vi "DSF.Shared.Configuration.Transfer.Set Channel Configurations.vi"(10 "Channel Configurations":refnum<class "DSF.Shared.Configuration.Channel.lvclass">[](array[class]), 11 "Transfer Configuration in":refnum<class "DSF.Shared.Configuration.Transfer.lvclass">) -> (3 "Transfer Configuration out":refnum<class "DSF.Shared.Configuration.Transfer.lvclass">)   [LabVIEW 2016, in "DSF.Shared.lvlib" / "DSF.Shared.Configuration.Transfer.lvclass"]
uses:
  DSF.Shared.Configuration.Transfer.lvclass
  Channel/DSF.Shared.Configuration.Channel.lvclass
  DSF.Shared.Configuration.Transfer.lvclass/DSF.Shared.Configuration.Transfer.ctl
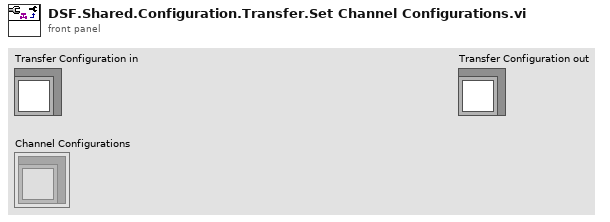
[diagram p1: front panel]
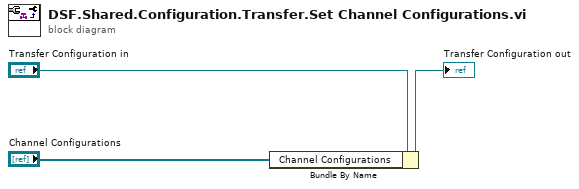
[diagram p0: block diagram]
diagram:
  n1 = Bundle By Name(cluster="Transfer Configuration in", "Channel Configurations"="Channel Configurations") -> (→"Transfer Configuration out":refnum<class "DSF.Shared.Configuration.Transfer.lvclass">)
